vi "PZT read position.vi"(3 "error in (no error)":errorcluster caption="错误输入（无错误）", 4 "Origin":dbl=5.0, 5 "Range":dbl=10.92, 6 "VISA resource name":refnum<visa-resource-name> caption="VISA资源名称") -> (0 "错误输出":errorcluster, 1 "Current Position （mm  /  °）":dbl, 2 "VISA资源名称输出":refnum<visa-resource-name>)   [LabVIEW 2019]
uses:
  <vilib>/Utility/error.llb/DialogType.ctl
panel:
  # "mm  /  °"
  # "mm  /  °"
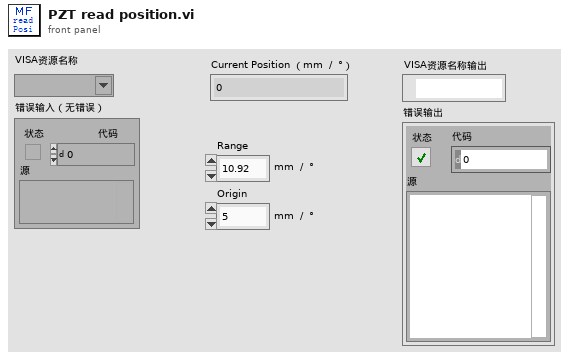
[diagram p1: front panel]
types:
  T1 = typedef "DialogType.ctl" = u16
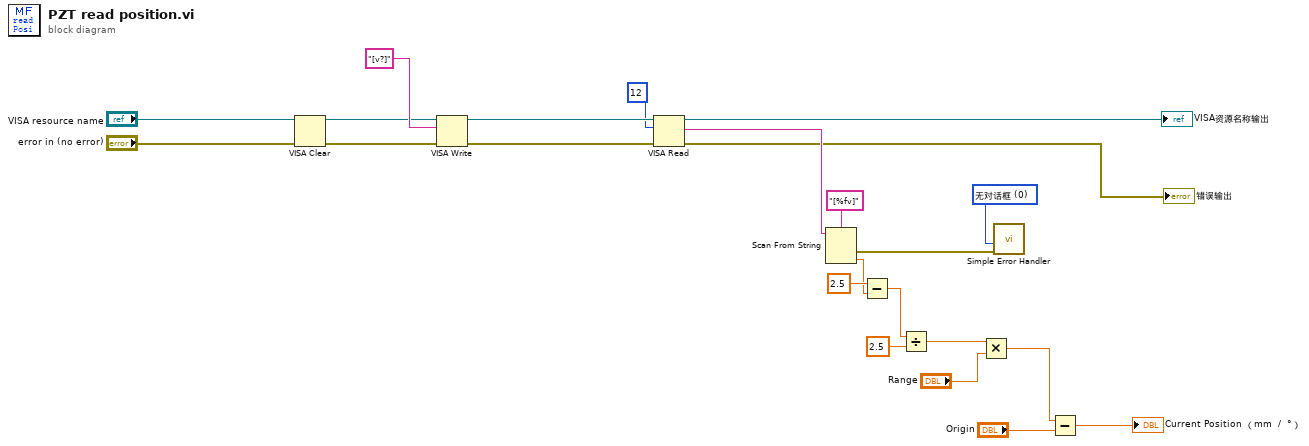
[diagram p0: block diagram]
diagram:
  w16 = T1 0 items=["无对话框", "确定信息", "继续或停止信息", "确定信息＋警告", "继续/停止+警告"] ("type of dialog (OK msg:1)")
  n1 = VISA Clear(VISA resource name="VISA resource name", error in (no error)="error in (no error)") -> (VISA resource name out=w11:refnum<visa-resource-name>, error out=w9:errorcluster)
  n2 = VISA Write(VISA resource name=w11, write buffer="[v?]" ("写入缓冲区"), error in (no error)=w9) -> (VISA resource name out=w22:refnum<visa-resource-name>, error out=w23:errorcluster)  [unwired: 1 out]
  n3 = VISA Read(VISA resource name=w22, byte count=u32 12 ("字节总数"), error in (no error)=w23) -> (VISA resource name out=→"VISA资源名称输出":refnum<visa-resource-name>, read buffer=w19:string, error out=→"错误输出":errorcluster)  [unwired: 1 out]
  n4 = Scan From String(format string="[%fv]" ("格式字符串"), input string=w19) -> (error out=w17:errorcluster, output 1=w2:dbl)  [unwired: 3 in, 2 out]
  n5 = Subtract(x=2.5, y=w2) -> (x-y=w1:dbl)
  n6 = Divide(x=w1, y=2.5) -> (x/y=w13:dbl)
  n7 = Multiply(x=w13, y="Range") -> (x*y=w5:dbl)
  n8 = call <vilib>:"Simple Error Handler.vi"("type of dialog (OK msg:1)"=w16, "error in (no error)"=w17) -> ()  [unwired: 3 in, 5 out]
  n9 = Subtract(x=w5, y="Origin") -> (x-y=→"Current Position （mm  /  °）":dbl)
